vi "Main-Strech DNA-OneDirectionOnly For OverStretching_YCC.vi"(4 "Avg points":i32=120, 5 "Save Data?":bool, 6 "Who's Data":enum16{"YCC", "PYW", "LCH", "YYH"}(ring), 7 "Set LaserPower (mV)":dbl=-2000.0 format="%0.2f", 8 "File name add to the end \n(laser power-height)":string="FA5180-h300", 9 "Record scan rate  (um/s)":dbl=4.0 format="%.3f", 10 "range  (um)":dbl=3.1 format="%.3f", 11 "T=X\nF=Y":bool=TRUE) -> (3 "Stage-QPD Graph":T4(graph))   [LabVIEW 2014]
uses:
  Main-Calibration/WLC fitting/SubVI/WLC-Fitting Cluster.ctl
  <vilib>/Analysis/baseanly.llb/Mean (DBL).vi
  <vilib>/Analysis/NI_AALBase.lvlib
panel:
  in  "Force offset":dbl=80.0
  in  "Length offset":dbl=700.0
  in  "Filter type":T1(ring)=enum."F+S-window avg"
  in  "trap height(nm)":dbl=300.0
  out "Laser Lock?":bool
  in  "xDNA cut outside":dbl=3000.0
  in  "Fitting Cluster 2":T2={"cr (um)"=0.0, "yr (V)"=0.0, "trap height(nm)"=0.0, "bead radius(nm)"=520.0, "Length offset"=0.0, "Upper Force(pN)"=0.0, "cr shift (nm)"=0.0, "yr shift (mV)"=0.0, "LaserPower (mW)"=0.0, "conversion factor (V/um)"=0.0, "Stiffness (pN/nm)"=0.0154, "xDNA cut outside"=0.0, "Lower Force(pN)"=5.0, "c for zbd"=0.0}
  out "True rate?":bool
  in  "no fec":bool=TRUE
  in  "Avg. time delay (ms)":dbl=18.0
  in  "Use avg delay?":bool=TRUE
  out "delay time between F and U (ms)":dbl
  out "initial QPD (V)":dbl format="%0.5f"
  in  "no Record scan rate  (um/s)":dbl=4.0
  out "Fold QPD Signal (V) 2":dbl[](array[numeric])
  out "Fold Stage Position (um) 2":dbl[](array[numeric])
  out "Folded-Force":dbl[](array[numeric])
  out "Folded-xDNA":dbl[](array[numeric])
  out "Unfolded-Force":dbl[](array[numeric])
  out "Unfolded-xDNA":dbl[](array[numeric])
  out "Filtered QPD Array":dbl[][](array[numeric])
  out "Filtered Stage Array":dbl[][](array[numeric])
  out "Save to File Name Indicator":string
  out "Save to Path Indicator":path
  out "initial position offset after move":dbl[](array[numeric])
  out "Avg. to Hz":dbl
  out "Fold QPD Signal (V)":dbl[](array[numeric])
  out "Unfold QPD Signal (V)":dbl[](array[numeric])
  out "Fold Stage Position (um)":dbl[](array[numeric])
  out "Unfold Stage Position (um)":dbl[](array[numeric])
  in  "Tab Control":T3(tab)
  out "Stage-QPD Graph 3":T4(graph)
  out "Stage-QPD Graph 2":T4(graph)
  out "Unfolded Graph":cluster{dbl[], dbl[]}(graph)
  out "Folded Graph":cluster{dbl[], dbl[]}(graph)
  out "Unfolded+Folded Graph":T5(graph)
  out "Trace direction":bool[](array[boolean])=[FALSE, TRUE, TRUE, FALSE]
  out "Real initial position (um)":dbl format="%0.5f"
  in  "Toward first ?\nT=+, F=-":bool
  in  "Record Mode \npath(1,2)":bool[](array[boolean])=[TRUE, TRUE, FALSE, FALSE]
  in  "Sampling rate":dbl=32000.0 format="%0.2f"
  # "range=3.1um & 4 um/s \nfor activead"
  # "avg delay= 33ms\n20181223 ·s¬°18ms"
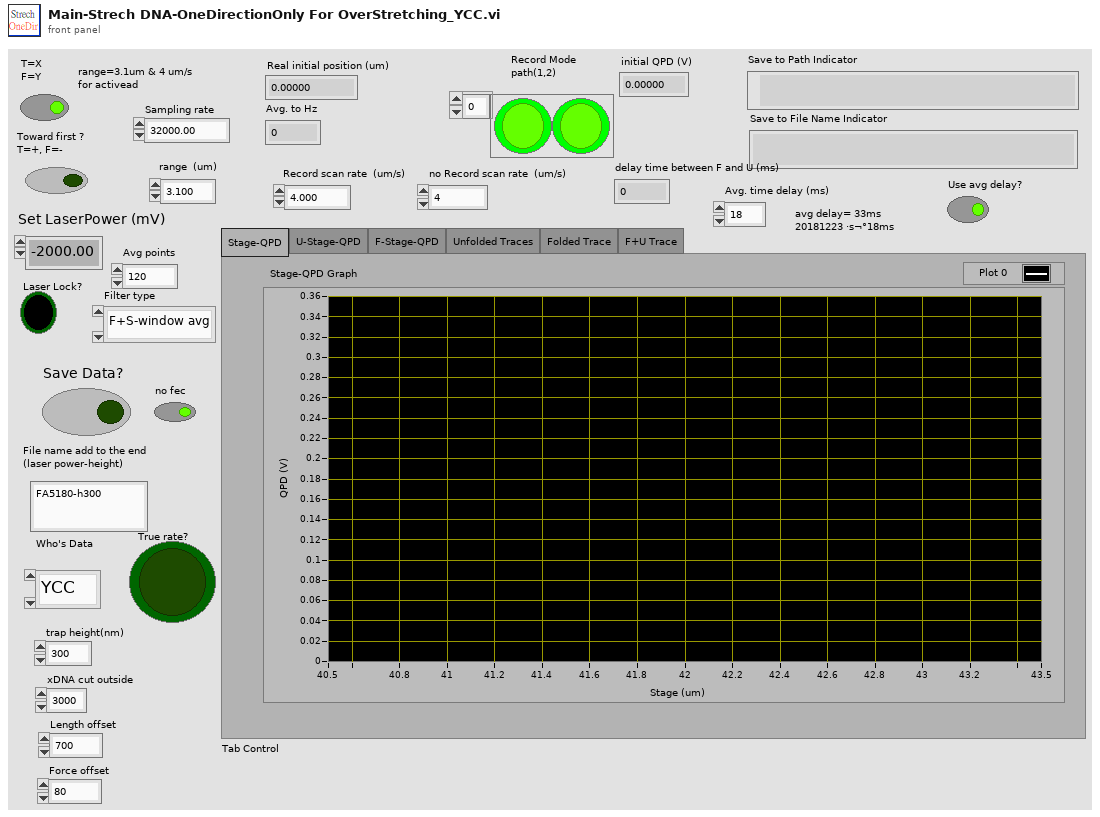
[diagram p1: front panel]
types:
  T1 = enum16{"Fixed-window avg", "Moving-window avg", "F+S-window avg", "S-G filter", "Fixed-window Median", "Moving-window Median "}
  T2 = typedef "WLC-Fitting Cluster.ctl" = cluster{"cr (um)":dbl, "yr (V)":dbl, "trap height(nm)":dbl, "bead radius(nm)":dbl, "Length offset":dbl, "Upper Force(pN)":dbl, "cr shift (nm)":dbl, "yr shift (mV)":dbl, "LaserPower (mW)":dbl, "conversion factor (V/um)":dbl, "Stiffness (pN/nm)":dbl, "xDNA cut outside":dbl, "Lower Force(pN)":dbl, "c for zbd":dbl}
  T3 = enum32{"Stage-QPD", "U-Stage-QPD", "F-Stage-QPD", "Unfolded Traces", "Folded Trace", "F+U Trace"}
  T4 = cluster{"Fold Stage Position (um)":dbl[], "Fold QPD Signal (V)":dbl[]}
  T5 = cluster{"Filtered Stage Array":dbl[], "Filtered QPD Array":dbl[]}[]
  T6 = enum16{"Custom", "Centering", "1000 mV", "4500 mV"}
  T7 = cluster{"Unfolded-xDNA":dbl[], "Unfolded-Force":dbl[]}
  T8 = cluster{"Folded-xDNA":dbl[], "Folded-Force":dbl[]}
  T9 = cluster{"Folded-xDNA":dbl[], "Folded-Force":dbl[]}[]
  T10 = cluster{"Unfold Stage Position (um)":dbl[], "Unfold QPD Signal (V)":dbl[]}
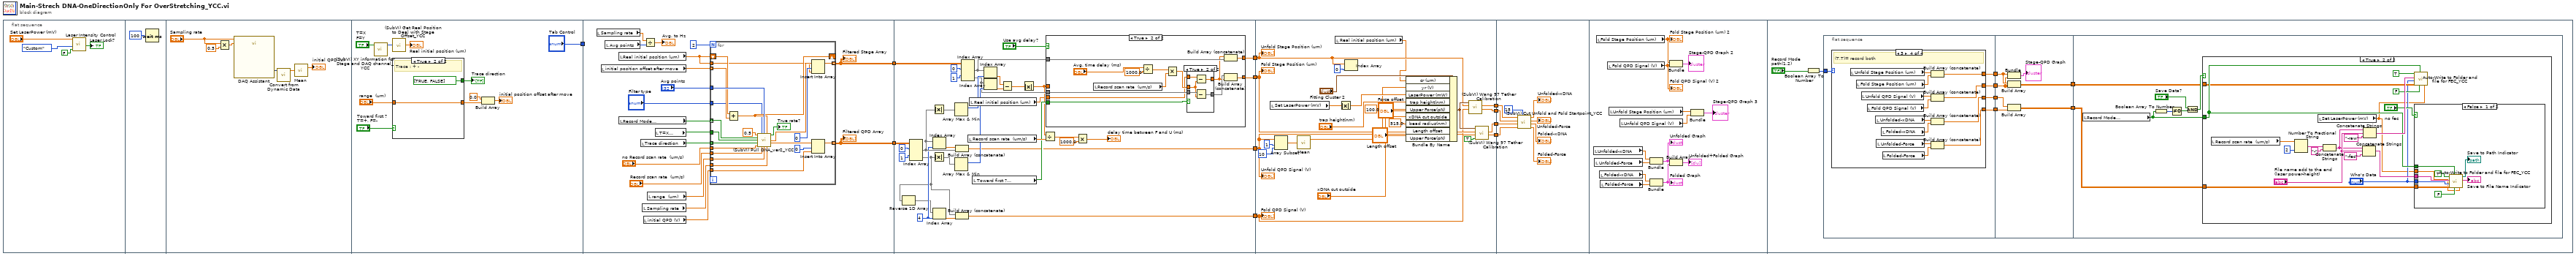
[diagram p0: block diagram]
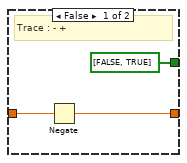
[diagram p2: hidden frame]
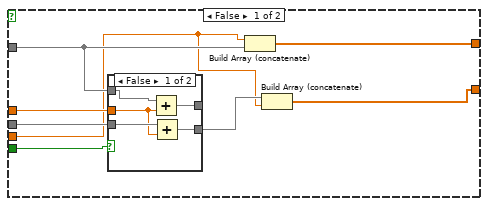
[diagram p3: hidden frame]
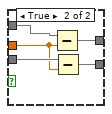
[diagram p4: hidden frame]
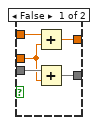
[diagram p5: hidden frame]
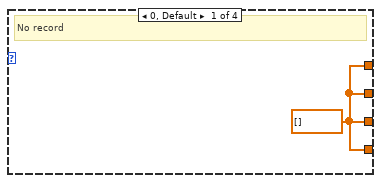
[diagram p6: hidden frame]
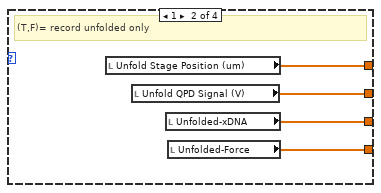
[diagram p7: hidden frame]
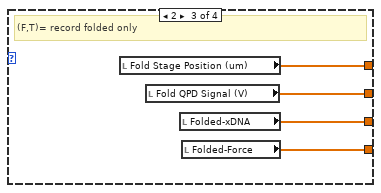
[diagram p8: hidden frame]
diagram:
  n1 = flat-sequence {
    tunnel: ["Tab Control"] -> w11
    tunnel: [w45] -> w5
    tunnel: [w44] -> w6
    tunnel: w11 -> [_]
    tunnel: w6 -> [w105]
    tunnel: w5 -> [w108]
    tunnel: [w90] -> w4
    tunnel: [w85] -> w3
    tunnel: [w84] -> w2
    tunnel: [w87] -> w1
    tunnel: [w175] -> w10
    tunnel: [w174] -> w9
    tunnel: [w173] -> w8
    tunnel: [w172] -> w7
    tunnel: w4 -> [w171]
    tunnel: w3 -> [w159]
    tunnel: w2 -> [w170]
    tunnel: w1 -> [w160]
    tunnel: w10 -> [w185]
    tunnel: w9 -> [w184]
    tunnel: w8 -> [w181]
    tunnel: w7 -> [w179]
    frame #0 {
      n2 = call "Laser Intensity Control.vi"("Close?"=FALSE, "Enum"=T6."Custom", "Intensity Control, 0~-7000 (mV)"="Set LaserPower (mV)") -> ("Laser Lock?"=→"Laser Lock?":bool)  [unwired: 4 in]
    }
    frame #1 {
      n3 = Wait (ms)(milliseconds to wait=u32 100) -> ()  [unwired: 1 out]
    }
    frame #2 {
      n4 = Multiply(x="Sampling rate", y=0.5) -> (x*y=w20:dbl)
      n5 = call "DAQ Assistant"("rate"="Sampling rate", "number of samples"=w20) -> ("data"=w19:dynamicdata)  [unwired: 15 in, 2 out]
      n6 = call "Convert from Dynamic Data"("Dynamic Data Type"=w19) -> ("Array"=w18:dbl[])  [unwired: 3 in]
      n7 = call-poly <vilib>:"Mean.vi"("X"=w18) -> ("mean"=→"initial QPD (V)":dbl)  [unwired: 1 out]
    }
    frame #3 {
      n8 = call "(SubVI) XY information for Stage and DAQ channel_YCC.vi"("T=X\nF=Y"="T=X\nF=Y") -> ("Axis"=w30:i32)  [unwired: 3 in, 1 out]
      n9 = call "(SubVI) Get Real Position to Deal with Stage Offset_YCC.vi"("Axis"=w30) -> ("Real Current Commanded position (um)"=→"Real initial position (um)":dbl)  [unwired: 3 in, 1 out]
      n10 = case shown="True" "Toward first ?\nT=+, F=-" {
        tunnel: [bool[] [FALSE, TRUE] bool[] [TRUE, FALSE]] -> w28
        tunnel: "range  (um)" -> [w34 w36]
        tunnel: [w33 w36] -> w23
        frame False {
          # "Trace : - +"
          n11 = Negate(x=w34) -> (-x=w33:dbl)
        }
        frame True {
          # "Trace : + -"
        }
      }
      "Trace direction" <- w28
      n12 = Build Array(0.0, w23) -> (→"initial position offset after move":dbl[])
    }
    frame #4 {
      n13 = local read "Sampling rate"() -> (w50:dbl)
      n14 = local read "initial position offset after move"() -> (w46:dbl[])
      n15 = local read "Avg points"() -> (w49:i32)
      n16 = local read "Real initial position (um)"() -> (w40:dbl)
      n17 = local read "Record Mode \npath(1,2)"() -> (w52:bool[])
      n18 = local read "Trace direction"() -> (w53:bool[])
      n19 = local read "Sampling rate"() -> (w41:dbl)
      n20 = local read "initial QPD (V)"() -> (w39:dbl)
      n21 = Divide(x=w50, y=w49) -> (x/y=→"Avg. to Hz":dbl)
      n22 = local read "range  (um)"() -> (w47:dbl)
      n23 = local read "T=X\nF=Y"() -> (w54:bool)
      n24 = for {
        N: 2 -> [_]
        tunnel: "Avg points" -> [w77]
        tunnel: w52 -> [w76] mode=indexing
        tunnel: w54 -> [w75]
        tunnel: w53 -> [w68] mode=indexing
        tunnel: w41 -> [w74]
        tunnel: "Record scan rate  (um/s)" -> [w73]
        tunnel: w47 -> [w72]
        tunnel: [w61] -> w45 mode=indexing
        tunnel: [w59] -> w44 mode=indexing
        shift-right: [w69] -> _
        shift-left: w40 -> [w70]
        tunnel: w46 -> [w71] mode=indexing
        tunnel: "no Record scan rate  (um/s)" -> [w67]
        tunnel: w40 -> [w62]
        tunnel: w39 -> [w60]
        tunnel: "Filter type" -> [w56]
        n25 = Add(x=w70, y=w71) -> (x+y=w69:dbl)
        n26 = call "(SubVI) Pull DNA_ver2_YCC.vi"("waiting time per point (ms)\nrange from 5ms to 0.167 ms"=0.5 ("waiting time per point (ms)\nrange from 5ms to 0.167 ms"), "Filter type"=w56, "Avg points"=w77, "Real initial position (um)"=w69, "Record?"=w76, "T=X\nF=Y"=w75, "Toward  ?\nT=+, F=-"=w68, "no Record scan rate  (um/s)"=w67, "Record scan rate  (um/s)"=w73, "range  (um)"=w72, "Sampling rate"=w74) -> ("True rate?"=→"True rate?":bool, "Filtered Stage Array"=w66:dbl[], "Filtered QPD Array"=w63:dbl[])  [unwired: 1 in, 1 out]
        n27 = Insert Into Array(array=w66, index=0, new element=w62) -> (w61:dbl[])
        n28 = Insert Into Array(array=w63, index=0, new element=w60) -> (w59:dbl[])
      }
      "Filtered Stage Array" <- w45
      "Filtered QPD Array" <- w44
    }
    frame #5 {
      w82 = 4 ("index")
      n29 = Index Array(array=w105, index (row) #1=0 ("index (row)"), index (row) #2=1 ("index (row)")) -> (element #1=w83:dbl[], element #2=w79:dbl[])  [unwired: 2 in]
      n30 = Reverse 1D Array(array=w79) -> (reversed array=w78:dbl[])
      n31 = Absolute Value(x=w83) -> (abs(x)=w104:dbl[])
      n32 = Absolute Value(x=w79) -> (abs(x)=w103:dbl[])
      n33 = Index Array(array=w83, index=w82) -> (element=w81:dbl)
      n34 = Index Array(array=w78, index=w82) -> (element=w80:dbl)
      n35 = Array Max & Min(array=w104) -> (max index (indices)=w100:i32)  [unwired: 3 out]
      n36 = Array Max & Min(array=w103) -> (max index (indices)=w99:i32)  [unwired: 3 out]
      n37 = Build Array (concatenate)(w81, w83) -> (w85:dbl[])
      n38 = Build Array (concatenate)(w79, w80) -> (w84:dbl[])
      n39 = Index Array(array=w108, index (row) #1=0 ("index (row)"), index (row) #2=1 ("index (row)")) -> (element #1=w88:dbl[], element #2=w92:dbl[])  [unwired: 2 in]
      n40 = local read "Record scan rate  (um/s)"() -> (w94:dbl)
      n41 = local read "Real initial position (um)"() -> (w86:dbl)
      n42 = local read "Toward first ?\nT=+, F=-"() -> (w93:bool)
      n43 = Index Array(array=w88, index=w100) -> (element=w102:dbl)
      n44 = Index Array(array=w92, index=w99) -> (element=w101:dbl)
      n45 = Subtract(x=w102, y=w101) -> (x-y=w95:dbl)
      n46 = Absolute Value(x=w95) -> (abs(x)=w91:dbl)
      n47 = Divide(x=w91, y=w94) -> (x/y=w98:dbl)
      n48 = case shown="True" "Use avg delay?" {
        tunnel: w93 -> [w118 w139]
        tunnel: w92 -> [w117 w140]
        tunnel: w91 -> [w116 _]
        tunnel: [w113 w130] -> w90
        tunnel: w88 -> [w112 w134]
        tunnel: [w115 w133] -> w87
        tunnel: w86 -> [w111 w129]
        frame False {
          n49 = case shown="False" w118 {
            tunnel: w117 -> [w123 w128]
            tunnel: w116 -> [w121 w126]
            tunnel: [w122 w127] -> w114
            tunnel: [w120 w125] -> _
            tunnel: w112 -> [w119 w124]
            frame False {
              n50 = Add(x=w119, y=w121) -> (x+y=w120:dbl[])
              n51 = Add(x=w123, y=w121) -> (x+y=w122:dbl[])
            }
            frame True {
              n52 = Subtract(x=w124, y=w126) -> (x-y=w125:dbl[])
              n53 = Subtract(x=w128, y=w126) -> (x-y=w127:dbl[])
            }
          }
          n54 = Build Array (concatenate)(w111, w112) -> (w115:dbl[])
          n55 = Build Array (concatenate)(w114, w111) -> (w113:dbl[])
        }
        frame True {
          n56 = local read "Record scan rate  (um/s)"() -> (w141:dbl)
          n57 = Divide(x="Avg. time delay (ms)", y=1000.0) -> (x/y=w136:dbl)
          n58 = Multiply(x=w136, y=w141) -> (x*y=w138:dbl)
          n59 = case shown="True" w139 {
            tunnel: w140 -> [w146 w151]
            tunnel: w138 -> [w143 w148]
            tunnel: [w145 w150] -> w132
            tunnel: w129 -> [w144 w149]
            tunnel: [w142 w147] -> w131
            frame False {
              n60 = Add(x=w144, y=w143) -> (x+y=w142:dbl)
              n61 = Add(x=w146, y=w143) -> (x+y=w145:dbl[])
            }
            frame True {
              n62 = Subtract(x=w149, y=w148) -> (x-y=w147:dbl)
              n63 = Subtract(x=w151, y=w148) -> (x-y=w150:dbl[])
            }
          }
          n64 = Build Array (concatenate)(w131, w134) -> (w133:dbl[])
          n65 = Build Array (concatenate)(w132, w131) -> (w130:dbl[])
        }
      }
      n66 = Multiply(x=w98, y=1000.0) -> (x*y=→"delay time between F and U (ms)":dbl)
    }
    frame #6 {
      n67 = local read "Set LaserPower (mV)"() -> (w164:dbl)
      n68 = Array Subset(array=w159, index=1, length=10) -> (w156:dbl[])
      n69 = call-poly <vilib>:"Mean.vi"("X"=w156) -> ("mean"=w155:dbl)  [unwired: 1 out]
      n70 = local read "Real initial position (um)"() -> (w152:dbl)
      n71 = Absolute Value(x=w164) -> (abs(x)=w163:dbl)
      n72 = Index Array(array=w160, index=0) -> ()  [unwired: 1 out]
      n73 = Bundle By Name(cluster="Fitting Cluster 2", "cr (um)"=w152, "yr (V)"=w155, "LaserPower (mW)"=w163, "trap height(nm)"="trap height(nm)", "Upper Force(pN)"=100.0 ("Force offset"), "xDNA cut outside"="xDNA cut outside", "bead radius(nm)"=515.0, "Length offset"="Length offset", "Upper Force(pN)"="Force offset") -> (w168:T2)
      n74 = call "(SubVI) Wang 97 Tether Calibration.vi"("QPD signal"=w159, "Stage Position"=w160, "Fitting Cluster"=w168) -> ("Force"=w174:dbl[], "xDNA"=w175:dbl[])  [unwired: 2 in, 1 out]
      n75 = call "(SubVI) Wang 97 Tether Calibration.vi"("X=T\nY=F"=TRUE ("X=T\nY=F"), "QPD signal"=w170, "Stage Position"=w171, "Fitting Cluster"=w168) -> ("Force"=w172:dbl[], "xDNA"=w173:dbl[])  [unwired: 1 in, 1 out]
      "Unfold Stage Position (um)" <- w160
      "Fold Stage Position (um)" <- w171
      "Unfold QPD Signal (V)" <- w159
      "Fold QPD Signal (V)" <- w170
    }
    frame #7 {
      n76 = call "(SubVI) Cut Unfold and Fold Startpoint_YCC.vi"("number to cut"=15, "Folded-Force in"=w179, "Folded-xDNA in"=w181, "Unfolded-Force"=w184, "Unfolded-xDNA"=w185) -> ("Folded-Force"=→"Folded-Force":dbl[], "Folded-xDNA"=→"Folded-xDNA":dbl[], "Unfolded-Force"=→"Unfolded-Force":dbl[], "Unfolded-xDNA"=→"Unfolded-xDNA":dbl[])  [unwired: 3 in]
    }
    frame #8 {
      n77 = local read "Unfolded-xDNA"() -> (w198:dbl[])
      n78 = local read "Unfolded-Force"() -> (w197:dbl[])
      n79 = local read "Fold Stage Position (um)"() -> (w190:dbl[])
      "Fold Stage Position (um) 2" <- w190
      n80 = local read "Folded-xDNA"() -> (w195:dbl[])
      n81 = local read "Folded-Force"() -> (w194:dbl[])
      n82 = local read "Fold QPD Signal (V)"() -> (w189:dbl[])
      "Fold QPD Signal (V) 2" <- w189
      n83 = local read "Unfold Stage Position (um)"() -> (w188:dbl[])
      n84 = local read "Unfold QPD Signal (V)"() -> (w187:dbl[])
      n85 = Bundle("Unfolded-xDNA"=w198, "Unfolded-Force"=w197) -> (w196:T7)  [unwired: 1 in]
      "Unfolded Graph" <- w196
      n86 = Bundle("Folded-xDNA"=w195, "Folded-Force"=w194) -> (w192:T8)  [unwired: 1 in]
      "Folded Graph" <- w192
      n87 = Bundle("Fold Stage Position (um)"=w190, "Fold QPD Signal (V)"=w189) -> (→"Stage-QPD Graph 2":T4)  [unwired: 1 in]
      n88 = Build Array(w196, w192) -> (→"Unfolded+Folded Graph":T9)
      n89 = Bundle("Unfold Stage Position (um)"=w188, "Unfold QPD Signal (V)"=w187) -> (→"Stage-QPD Graph 3":T10)  [unwired: 1 in]
    }
    frame #9 {
      n90 = Boolean Array To Number(Boolean array="Record Mode \npath(1,2)") -> (number=w205:u32)
      n91 = flat-sequence {
        tunnel: w205 -> [w209]
        tunnel: [w211] -> w204
        tunnel: [w210] -> w203
        tunnel: [w208] -> w201
        tunnel: [w207] -> w200
        tunnel: w204 -> [w235]
        tunnel: w203 -> [w234]
        tunnel: [w239] -> w202
        tunnel: w201 -> [w238]
        tunnel: w200 -> [w237]
        tunnel: [w236] -> w199
        tunnel: w202 -> [w243]
        tunnel: w199 -> [w240]
        frame #0 {
          n92 = case shown="3" w209 {
            tunnel: [w212 w216 w220 w228] -> w211
            tunnel: [w212 w215 w219 w227] -> w210
            tunnel: [w212 w214 w218 w222] -> w208
            tunnel: [w212 w213 w217 w221] -> w207
            frame 0, Default {
              w212 = dbl[] [] ("Fold Stage Position (um)")
              # "No record"
            }
            frame 1 {
              # "(T,F)= record unfolded only"
              n93 = local read "Unfold Stage Position (um)"() -> (w216:dbl[])
              n94 = local read "Unfold QPD Signal (V)"() -> (w215:dbl[])
              n95 = local read "Unfolded-xDNA"() -> (w214:dbl[])
              n96 = local read "Unfolded-Force"() -> (w213:dbl[])
            }
            frame 2 {
              # "(F,T)= record folded only"
              n97 = local read "Fold Stage Position (um)"() -> (w220:dbl[])
              n98 = local read "Fold QPD Signal (V)"() -> (w219:dbl[])
              n99 = local read "Folded-xDNA"() -> (w218:dbl[])
              n100 = local read "Folded-Force"() -> (w217:dbl[])
            }
            frame 3 {
              # "(T,T)= record both"
              n101 = local read "Unfold Stage Position (um)"() -> (w232:dbl[])
              n102 = local read "Fold Stage Position (um)"() -> (w231:dbl[])
              n103 = local read "Unfold QPD Signal (V)"() -> (w230:dbl[])
              n104 = local read "Fold QPD Signal (V)"() -> (w229:dbl[])
              n105 = local read "Unfolded-xDNA"() -> (w226:dbl[])
              n106 = local read "Unfolded-Force"() -> (w224:dbl[])
              n107 = local read "Folded-xDNA"() -> (w225:dbl[])
              n108 = local read "Folded-Force"() -> (w223:dbl[])
              n109 = Build Array (concatenate)(w232, w231) -> (w228:dbl[])
              n110 = Build Array (concatenate)(w230, w229) -> (w227:dbl[])
              n111 = Build Array (concatenate)(w226, w225) -> (w222:dbl[])
              n112 = Build Array (concatenate)(w224, w223) -> (w221:dbl[])
            }
          }
        }
        frame #1 {
          n113 = Bundle("Fold Stage Position (um)"=w235, "Fold QPD Signal (V)"=w234) -> (→"Stage-QPD Graph":T4)  [unwired: 1 in]
          n114 = Build Array(w235, w234) -> (w239:dbl[][])
          n115 = Build Array(w238, w237) -> (w236:dbl[][])
        }
        frame #2 {
          n116 = local read "Record Mode \npath(1,2)"() -> (w241:bool[])
          n117 = Boolean Array To Number(Boolean array=w241) -> (number=w242:u32)
          n118 = Not Equal To 0?(x=w242) -> (x != 0?=w245:bool)
          n119 = And(x="Save Data?", y=w245) -> (x .and. y?=w244:bool)
          n120 = case shown="True" w244 {
            tunnel: w243 -> [_ w256]
            tunnel: w241 -> [_ w258]
            tunnel: w240 -> [_ w257]
            frame False {
            }
            frame True {
              n121 = local read "Record scan rate  (um/s)"() -> (w252:dbl)
              n122 = Number To Fractional String(number=w252, precision (6)=i16 2) -> (F-format string=w253:string)  [unwired: 2 in]
              n123 = local read "Set LaserPower (mV)"() -> (w247:dbl)
              n124 = Concatenate Strings(w253, "-") -> (w251:string)
              n125 = Concatenate Strings(w251, "File name add to the end \n(laser power-height)", "-fec" ("string")) -> (w262:string)
              n126 = Concatenate Strings(w251, "File name add to the end \n(laser power-height)", "-raw" ("string")) -> (w259:string)
              n127 = call "Auto-Write to Folder and file for FEC_YCC.vi"("Current PD (mV)"=w247, "Centering data?"=FALSE, "Record Mode \npath(1,2)"=w258, "data to be saved"=w256, "Who's Data"="Who's Data", "File name add to the end \n(height)"=w259, "Save?"=TRUE) -> ()  [unwired: 1 in, 2 out]
              n128 = case shown="False" "no fec" {
                tunnel: w262 -> [w270 _]
                tunnel: w258 -> [w269 _]
                tunnel: w257 -> [w268 _]
                tunnel: "Who's Data" -> [w266 _]
                tunnel: w247 -> [w265 _]
                frame False {
                  n129 = call "Auto-Write to Folder and file for FEC_YCC.vi"("Current PD (mV)"=w265, "Centering data?"=FALSE, "Record Mode \npath(1,2)"=w269, "data to be saved"=w268, "Who's Data"=w266, "File name add to the end \n(height)"=w270, "Save?"=TRUE) -> ("Save to File Name"=→"Save to File Name Indicator":string, "Save to Path"=→"Save to Path Indicator":path)  [unwired: 1 in]
                }
                frame True {
                }
              }
            }
          }
        }
      }
    }
  }
